vi "Read Local Tool Cfg XML File.vi"(8 "error in":errorcluster) -> (0 "error out":errorcluster, 1 "Tool Config":T1={"Tool Type"=0, "Tool SN"=0, "Tool Block"={"Encoder Size"=0, "Encoder Scale"=0, "Encoder Offset"=0, "MaxEncoder"=0, "MinEncoder"=0, "Start Delay"=0.0, "Tool Face Ref"=0.0}, "Motor Block"={"MinMotor Speed"=0, "MaxMotor Speed"=0, "Homing Speed"=90, "Jog Speed"=90, "Inspect Speed"=90, "VBlk Speed"=90, "CleaningPos"=0, "Safe Zone"=0, "Has Motor"=FALSE, "Use Home Index"=FALSE}, "Verification Block"={"Angle"=90.0, "FlankLength1"=0.0, "FlankLength2"=0.0, "Location"=0.0, "Serial Number"=0}, "Probe Block"={"nProbes"=0, "Probe Param Array"=[]}} {"Probe Block"."Probe Param Array"."Sensor Block"."SensorCfgParams Array"."CalibrCoefArray" format="%#.12g"}, 2 "Config Cluster Version":string, 3 "Product Name":string, 4 "XML File Path":path, 5 "Success":bool)   [LabVIEW 2015, in "Tool Cfg.lvlib"]
uses:
  Tool Cfg.lvlib
  _Configuration Cluster_v3--typedef.ctl
  _Tool Block Cluster_v3--typedef.ctl
  _Motor Block Cluster_v2--typedef.ctl
  _Verification Blk Cluster--typedef.ctl
  _ProbeConfigParams Cluster--typedef.ctl
  _Sensor Block Cluster--typedef.ctl
  _SensorConfigParams Cluster--typedef.ctl
  <vilib>/Utility/xml.llb/Read From XML File(array).vi
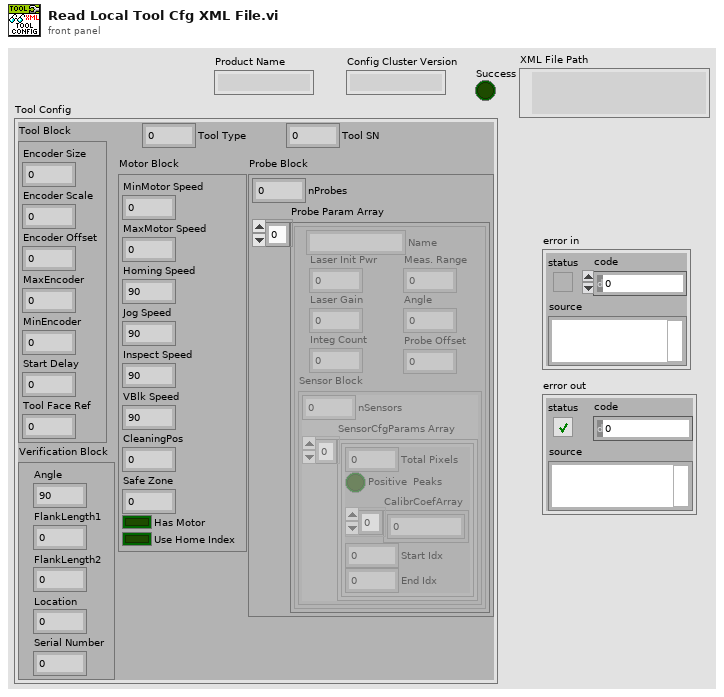
[diagram p1: front panel]
types:
  T1 = typedef "Tool Cfg.lvlib/_Configuration Cluster_v3--typedef.ctl" = cluster{"Tool Type":u16, "Tool SN":u16, "Tool Block":T2, "Motor Block":T3, "Verification Block":T4, "Probe Block":cluster{"nProbes":u16, "Probe Param Array":T5[]}}
  T2 = typedef "Tool Cfg.lvlib/_Tool Block Cluster_v3--typedef.ctl" = cluster{"Encoder Size":u16, "Encoder Scale":u32, "Encoder Offset":i32, "MaxEncoder":i32, "MinEncoder":i32, "Start Delay":sgl, "Tool Face Ref":sgl}
  T3 = typedef "Tool Cfg.lvlib/_Motor Block Cluster_v2--typedef.ctl" = cluster{"MinMotor Speed":u16, "MaxMotor Speed":u16, "Homing Speed":u16, "Jog Speed":u16, "Inspect Speed":u16, "VBlk Speed":u16, "CleaningPos":i32, "Safe Zone":i32, "Has Motor":bool, "Use Home Index":bool}
  T4 = typedef "Tool Cfg.lvlib/_Verification Blk Cluster--typedef.ctl" = cluster{"Angle":sgl, "FlankLength1":sgl, "FlankLength2":sgl, "Location":sgl, "Serial Number":u16}
  T5 = typedef "Tool Cfg.lvlib/_ProbeConfigParams Cluster--typedef.ctl" = cluster{"Name":string, "Laser Init Pwr":u16, "Laser Gain":u8, "Integ Count":u16, "Meas. Range":sgl, "Angle":sgl, "Probe Offset":sgl, "Sensor Block":T6}
  T6 = typedef "Tool Cfg.lvlib/_Sensor Block Cluster--typedef.ctl" = cluster{"nSensors":u16, "SensorCfgParams Array":T7[]}
  T7 = typedef "Tool Cfg.lvlib/_SensorConfigParams Cluster--typedef.ctl" = cluster{"Total Pixels":u16, "Positive  Peaks":bool, "CalibrCoefArray":dbl[], "Start Idx":u16, "End Idx":u16}
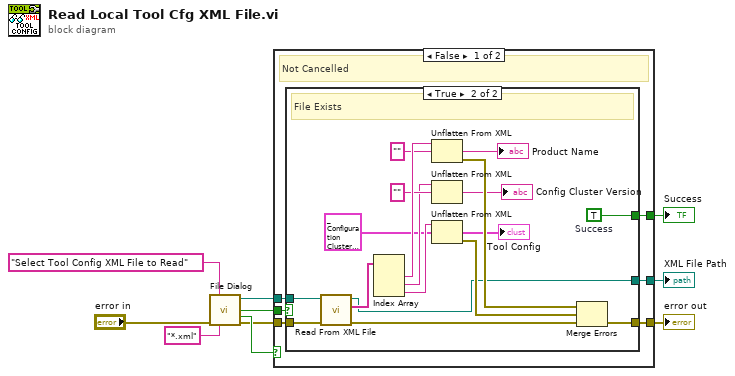
[diagram p0: block diagram]
diagram:
  n1 = call "File Dialog"("prompt"="Select Tool Config XML File to Read", "error in"="error in", "pattern (all files)"="*.xml") -> ("selected path"=w6:path, "exists"=w8:bool, "cancelled"=w7:bool, "error out"=w5:errorcluster)  [unwired: 9 in]
  n2 = case shown="False" w7 {
    tunnel: w8 -> [w16 _]
    tunnel: w6 -> [w15 _]
    tunnel: w5 -> [w14 w36]
    tunnel: [w13 w36] -> w4
    tunnel: [w12 _] -> w2
    tunnel: [w11 _] -> w1
    frame False {
      # "Not Cancelled"
      n3 = case shown="True" w16 {
        tunnel: w15 -> [_ w35]
        tunnel: w14 -> [w17 w34]
        tunnel: [w17 w26] -> w13
        tunnel: [_ w25] -> w12
        tunnel: [_ w20] -> w11
        frame False {
          # "File does not exist"
        }
        frame True {
          w25 = TRUE  # Success
          # "File Exists"
          n4 = call-poly <vilib>:"Read From XML File.vi"("error in (no error)"=w34, "XML File Path"=w35) -> ("error out"=w29:errorcluster, "XML Elements"=w33:string[], "XML File Path(duplicate)"=w20:path)  [unwired: 7 in]
          n5 = Index Array(array=w33) -> (element #1=w32:string, element #2=w22:string, element #3=w21:string)  [unwired: 3 in]
          n6 = Unflatten From XML(xml string=w32, type="") -> (value=→"Product Name":string, error out=w27:errorcluster)  [unwired: 1 in]
          n7 = Unflatten From XML(xml string=w22, type="") -> (value=→"Config Cluster Version":string)  [unwired: 1 in, 1 out]
          n8 = Unflatten From XML(xml string=w21, type=T1 {"Tool Type"=0, "Tool SN"=0, "Tool Block"={"Encoder Size"=0, "Encoder Scale"=0, "Encoder Offset"=0, "MaxEncoder"=0, "MinEncoder"=0, "Start Delay"=0.0, "Tool Face Ref"=0.0}, "Motor Block"={"MinMotor Speed"=0, "MaxMotor Speed"=0, "Homing Speed"=90, "Jog Speed"=90, "Inspect Speed"=90, "VBlk Speed"=90, "CleaningPos"=0, "Safe Zone"=0, "Has Motor"=FALSE, "Use Home Index"=FALSE}, "Verification Block"={"Angle"=90.0, "FlankLength1"=0.0, "FlankLength2"=0.0, "Location"=0.0, "Serial Number"=0}, "Probe Block"={"nProbes"=0, "Probe Param Array"=[]}} ("_Tool Config Cluster_v3--typedef")) -> (value=→"Tool Config":T1, error out=w28:errorcluster)  [unwired: 1 in]
          n9 = Merge Errors(w27, w28, w29) -> (w26:errorcluster)
        }
      }
    }
    frame True {
      # "Cancelled"
    }
  }
  "error out" <- w4
  "Success" <- w2
  "XML File Path" <- w1
